vi "Player Info.vi"(11 "Fortress In":refnum<class "Fortress.lvclass">) -> (0 "Defeat Speech":string, 1 "Victory Speech":string, 2 "Name":string, 3 "Fortress Out":refnum<class "Fortress.lvclass">)   [LabVIEW 2015, in "Fortress.lvclass"]
uses:
  Fortress.lvclass
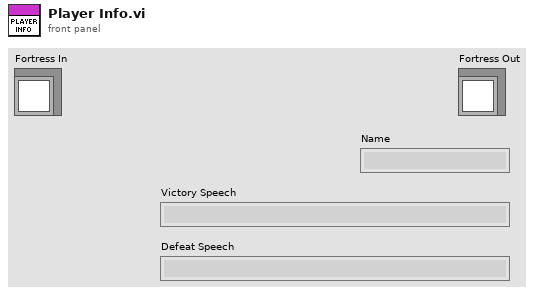
[diagram p1: front panel]
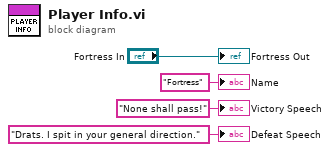
[diagram p0: block diagram]
diagram:
  "Fortress Out" <- "Fortress In"
  "Name" <- "Fortress" ("Name")
  "Victory Speech" <- "None shall pass!" ("Victory Speech")
  "Defeat Speech" <- "Drats. I spit in your general direction." ("Defeat Speech")
